vi "Anritsu_MT8852B_YYLL_ClearBuff.vi"(8 "error IO":errorcluster, 11 "VISA resource name":refnum<visa-resource-name>) -> (0 "error IO 2":errorcluster, 1 "BUFFString":string, 3 "VISA resource name 2":refnum<visa-resource-name>)   [LabVIEW 2017]
panel:
  # "#yyll 因为自带终止符的原因，\n所以需要暴力清除缓存-ok\n确保发送后收到是最新的-!?"
  # "MT8852B"
  # "Anritsu"
  # "YYLL"
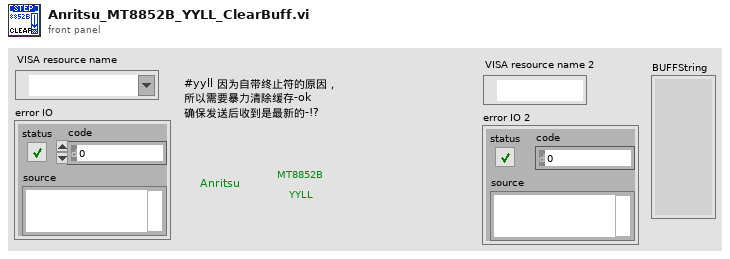
[diagram p1: front panel]
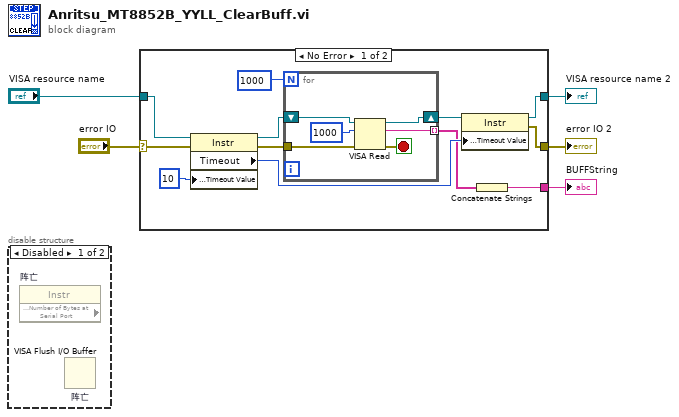
[diagram p0: block diagram]
diagram:
  n1 = disable-structure shown="Disabled" {
    frame Disabled {
      n2 = property on="阵亡" class="Instr" props=["Serial Settings:Number of Bytes at Serial Port"]() -> ()  [unwired: 2 in, 3 out]
      n3 = VISA Flush I/O Buffer "阵亡"() -> ()  [unwired: 3 in, 2 out]
    }
    frame Enabled {
    }
  }
  n4 = case shown="No Error" "error IO" {
    selector: "error IO" -> [w10 w24]
    tunnel: "VISA resource name" -> [w16 w25]
    tunnel: [w11 w25] -> w4
    tunnel: [w9 w24] -> w2
    tunnel: [w6 _] -> w1
    frame No Error {
      n5 = property class="Instr"(reference=w16, error in=w10, "General Settings:Timeout Value"=u32 10) -> (reference out=w15:refnum<visa-resource-name>, error out=w14:errorcluster, "Timeout"=w12:u32)
      n6 = for {
        N: 1000 -> [_]
        tunnel: w14 -> [w21]
        shift-right: [w20] -> w13
        shift-left: w15 -> [w22]
        tunnel: [w18] -> w7 mode=indexing
        stop <- w19 stop-if-true
        n7 = VISA Read(VISA resource name=w22, byte count=u32 1000 ("byte count (0)"), error in (no error)=w21) -> (VISA resource name out=w20:refnum<visa-resource-name>, read buffer=w18:string, error out=w19:errorcluster)  [unwired: 1 out]
      }
      n8 = property class="Instr"(reference=w13, "General Settings:Timeout Value"=w12) -> (reference out=w11:refnum<visa-resource-name>, error out=w9:errorcluster)  [unwired: 1 in]
      n9 = Concatenate Strings(w7) -> (w6:string)
    }
    frame Error {
    }
  }
  "VISA resource name 2" <- w4
  "error IO 2" <- w2
  "BUFFString" <- w1
